vi "Изменение коэффициентов3.vi"(0 "VISA Refnum in":refnum<visa-resource-name>, 1 "error in (no error)":errorcluster, 2 "f_cut_diff_vel_xy b":bool, 3 "KP_Pos_xy b":bool, 4 "KD_Vel_alt b":bool, 5 "KD_Vel_alt":dbl, 6 "f_cut_err_vel_xy":dbl, 7 "KI_Acc_alt b":bool, 8 "KD_Vel_xy":dbl, 9 "KP_Pos_xy":dbl, 10 "f_cut_err_vel_xy b":bool, 11 "f_cut_diff_vel_xy":dbl, 12 "KD_Vel_xy":bool, 13 "KP_Vel_xy b":bool, 14 "KI_Vel_xy":dbl, 15 "f_cut_diff_vel_alt":dbl, 16 "KI_Vel_xy b":bool, 17 "f_cut_diff_vel_alt b":bool, 20 "KI_Acc_alt":dbl, 21 "KD_Acc_alt b":bool, 23 "KP_Vel_xy":dbl, 24 "KD_Acc_alt":dbl, 25 "f_cut_diff_acc_alt b":bool, 27 "f_cut_diff_acc_alt":dbl) -> ()   [LabVIEW 2013]
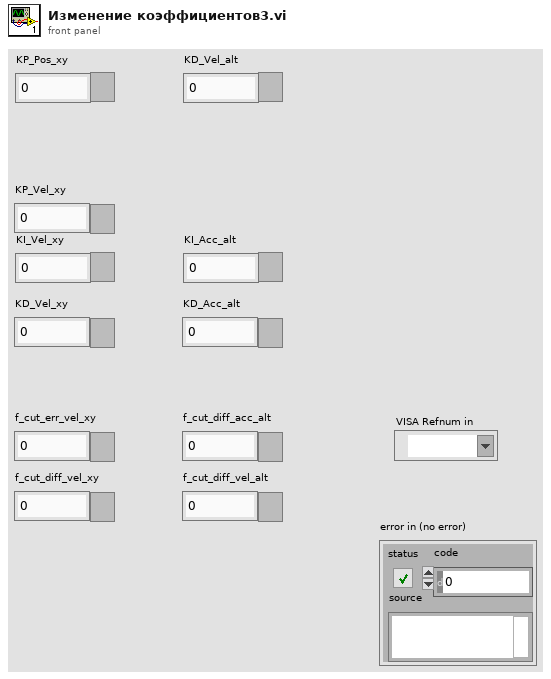
[diagram p1: front panel]
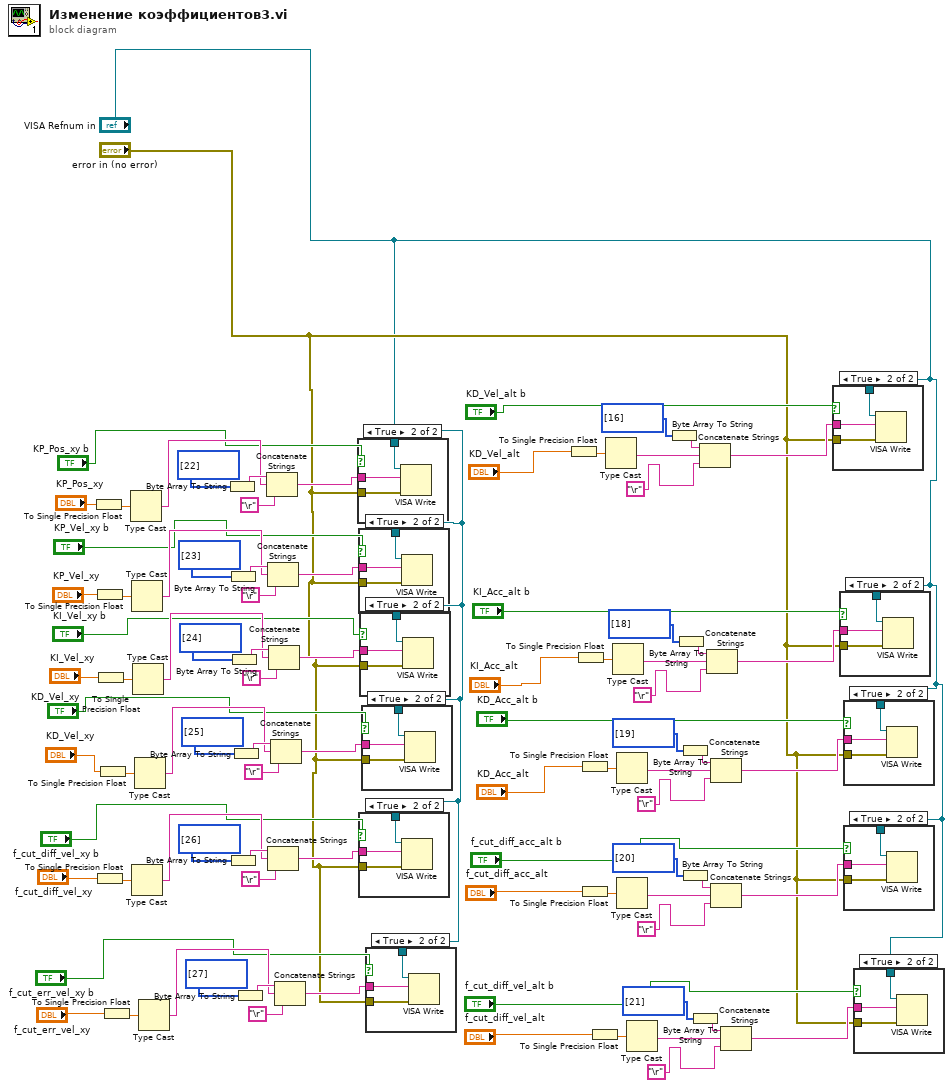
[diagram p0: block diagram]
diagram:
  n1 = To Single Precision Float(number="KP_Pos_xy") -> (single precision float=w46:sgl)
  n2 = To Single Precision Float(number="KP_Vel_xy") -> (single precision float=w38:sgl)
  n3 = To Single Precision Float(number="f_cut_diff_vel_xy") -> (single precision float=w14:sgl)
  n4 = To Single Precision Float(number="KI_Vel_xy") -> (single precision float=w30:sgl)
  n5 = To Single Precision Float(number="KD_Vel_xy") -> (single precision float=w22:sgl)
  n6 = To Single Precision Float(number="f_cut_err_vel_xy") -> (single precision float=w6:sgl)
  n7 = Type Cast(x=w46) -> (*(type *) &x=w45:string)  [unwired: 1 in]
  n8 = Type Cast(x=w38) -> (*(type *) &x=w37:string)  [unwired: 1 in]
  n9 = Type Cast(x=w14) -> (*(type *) &x=w13:string)  [unwired: 1 in]
  n10 = Type Cast(x=w30) -> (*(type *) &x=w29:string)  [unwired: 1 in]
  n11 = Type Cast(x=w22) -> (*(type *) &x=w21:string)  [unwired: 1 in]
  n12 = Type Cast(x=w6) -> (*(type *) &x=w5:string)  [unwired: 1 in]
  n13 = Byte Array To String(unsigned byte array=u8[] [22]) -> (string=w50:string)
  n14 = Byte Array To String(unsigned byte array=u8[] [23]) -> (string=w42:string)
  n15 = Byte Array To String(unsigned byte array=u8[] [26]) -> (string=w18:string)
  n16 = Byte Array To String(unsigned byte array=u8[] [24]) -> (string=w34:string)
  n17 = Byte Array To String(unsigned byte array=u8[] [25]) -> (string=w26:string)
  n18 = Byte Array To String(unsigned byte array=u8[] [27]) -> (string=w10:string)
  n19 = Concatenate Strings(w50, w45, "\r") -> (w48:string)
  n20 = Concatenate Strings(w42, w37, "\r") -> (w40:string)
  n21 = Concatenate Strings(w18, w13, "\r") -> (w16:string)
  n22 = Concatenate Strings(w34, w29, "\r") -> (w32:string)
  n23 = Concatenate Strings(w26, w21, "\r") -> (w24:string)
  n24 = Concatenate Strings(w10, w5, "\r") -> (w8:string)
  n25 = case shown="True" "KP_Pos_xy b" {
    tunnel: w48 -> [_ w93]
    tunnel: "VISA Refnum in" -> [_ w92]
    tunnel: "error in (no error)" -> [_ w91]
    frame False {
    }
    frame True {
      n26 = VISA Write(VISA resource name=w92, write buffer=w93, error in (no error)=w91) -> ()  [unwired: 3 out]
    }
  }
  n27 = case shown="True" "KP_Vel_xy b" {
    tunnel: w40 -> [_ w96]
    tunnel: "VISA Refnum in" -> [_ w95]
    tunnel: "error in (no error)" -> [_ w94]
    frame False {
    }
    frame True {
      n28 = VISA Write(VISA resource name=w95, write buffer=w96, error in (no error)=w94) -> ()  [unwired: 3 out]
    }
  }
  n29 = case shown="True" "f_cut_diff_vel_xy b" {
    tunnel: w16 -> [_ w99]
    tunnel: "VISA Refnum in" -> [_ w98]
    tunnel: "error in (no error)" -> [_ w97]
    frame False {
    }
    frame True {
      n30 = VISA Write(VISA resource name=w98, write buffer=w99, error in (no error)=w97) -> ()  [unwired: 3 out]
    }
  }
  n31 = case shown="True" "KI_Vel_xy b" {
    tunnel: w32 -> [_ w102]
    tunnel: "VISA Refnum in" -> [_ w101]
    tunnel: "error in (no error)" -> [_ w100]
    frame False {
    }
    frame True {
      n32 = VISA Write(VISA resource name=w101, write buffer=w102, error in (no error)=w100) -> ()  [unwired: 3 out]
    }
  }
  n33 = case shown="True" "KD_Vel_xy" {
    tunnel: w24 -> [_ w105]
    tunnel: "VISA Refnum in" -> [_ w104]
    tunnel: "error in (no error)" -> [_ w103]
    frame False {
    }
    frame True {
      n34 = VISA Write(VISA resource name=w104, write buffer=w105, error in (no error)=w103) -> ()  [unwired: 3 out]
    }
  }
  n35 = case shown="True" "f_cut_err_vel_xy b" {
    tunnel: w8 -> [_ w108]
    tunnel: "VISA Refnum in" -> [_ w107]
    tunnel: "error in (no error)" -> [_ w106]
    frame False {
    }
    frame True {
      n36 = VISA Write(VISA resource name=w107, write buffer=w108, error in (no error)=w106) -> ()  [unwired: 3 out]
    }
  }
  n37 = To Single Precision Float(number="KD_Vel_alt") -> (single precision float=w86:sgl)
  n38 = To Single Precision Float(number="KI_Acc_alt") -> (single precision float=w80:sgl)
  n39 = To Single Precision Float(number="KD_Acc_alt") -> (single precision float=w74:sgl)
  n40 = To Single Precision Float(number="f_cut_diff_acc_alt") -> (single precision float=w62:sgl)
  n41 = To Single Precision Float(number="f_cut_diff_vel_alt") -> (single precision float=w56:sgl)
  n42 = Type Cast(x=w86) -> (*(type *) &x=w85:string)  [unwired: 1 in]
  n43 = Type Cast(x=w80) -> (*(type *) &x=w79:string)  [unwired: 1 in]
  n44 = Type Cast(x=w74) -> (*(type *) &x=w73:string)  [unwired: 1 in]
  n45 = Type Cast(x=w62) -> (*(type *) &x=w61:string)  [unwired: 1 in]
  n46 = Type Cast(x=w56) -> (*(type *) &x=w55:string)  [unwired: 1 in]
  n47 = Byte Array To String(unsigned byte array=u8[] [16]) -> (string=w90:string)
  n48 = Byte Array To String(unsigned byte array=u8[] [18]) -> (string=w84:string)
  n49 = Byte Array To String(unsigned byte array=u8[] [19]) -> (string=w78:string)
  n50 = Byte Array To String(unsigned byte array=u8[] [20]) -> (string=w66:string)
  n51 = Byte Array To String(unsigned byte array=u8[] [21]) -> (string=w60:string)
  n52 = Concatenate Strings(w90, w85, "\r") -> (w88:string)
  n53 = Concatenate Strings(w84, w79, "\r") -> (w82:string)
  n54 = Concatenate Strings(w78, w73, "\r") -> (w76:string)
  n55 = Concatenate Strings(w66, w61, "\r") -> (w64:string)
  n56 = Concatenate Strings(w60, w55, "\r") -> (w58:string)
  n57 = case shown="True" "KD_Vel_alt b" {
    tunnel: w88 -> [_ w111]
    tunnel: "VISA Refnum in" -> [_ w110]
    tunnel: "error in (no error)" -> [_ w109]
    frame False {
    }
    frame True {
      n58 = VISA Write(VISA resource name=w110, write buffer=w111, error in (no error)=w109) -> ()  [unwired: 3 out]
    }
  }
  n59 = case shown="True" "KI_Acc_alt b" {
    tunnel: w82 -> [_ w114]
    tunnel: "VISA Refnum in" -> [_ w113]
    tunnel: "error in (no error)" -> [_ w112]
    frame False {
    }
    frame True {
      n60 = VISA Write(VISA resource name=w113, write buffer=w114, error in (no error)=w112) -> ()  [unwired: 3 out]
    }
  }
  n61 = case shown="True" "KD_Acc_alt b" {
    tunnel: w76 -> [_ w117]
    tunnel: "VISA Refnum in" -> [_ w116]
    tunnel: "error in (no error)" -> [_ w115]
    frame False {
    }
    frame True {
      n62 = VISA Write(VISA resource name=w116, write buffer=w117, error in (no error)=w115) -> ()  [unwired: 3 out]
    }
  }
  n63 = case shown="True" "f_cut_diff_acc_alt b" {
    tunnel: w64 -> [_ w120]
    tunnel: "VISA Refnum in" -> [_ w119]
    tunnel: "error in (no error)" -> [_ w118]
    frame False {
    }
    frame True {
      n64 = VISA Write(VISA resource name=w119, write buffer=w120, error in (no error)=w118) -> ()  [unwired: 3 out]
    }
  }
  n65 = case shown="True" "f_cut_diff_vel_alt b" {
    tunnel: w58 -> [_ w123]
    tunnel: "VISA Refnum in" -> [_ w122]
    tunnel: "error in (no error)" -> [_ w121]
    frame False {
    }
    frame True {
      n66 = VISA Write(VISA resource name=w122, write buffer=w123, error in (no error)=w121) -> ()  [unwired: 3 out]
    }
  }
